vi "Filter Event Data.vi"(8 "error in (no error)":errorcluster, 10 "EventFilter Reference":T1, 11 "ListboxEditCellMsg In":refnum<class "ListboxEditCellMsg.lvclass">) -> (0 "error out":errorcluster, 2 "Discard?":bool, 3 "ListboxEditCellMsg Out":refnum<class "ListboxEditCellMsg.lvclass">)   [LabVIEW 2020, in "MVA Framework.lvlib" / "ActorEvents.lvlib" / "ListboxEditCellMsg.lvclass"]
uses:
  ListboxEditCellMsg.lvclass
  IEventFilter/EventFilter Reference.ctl
  IEventFilter/IEventFilter.lvclass
  ListboxEditCellMsg.lvclass/ListboxEditCellMsg.ctl
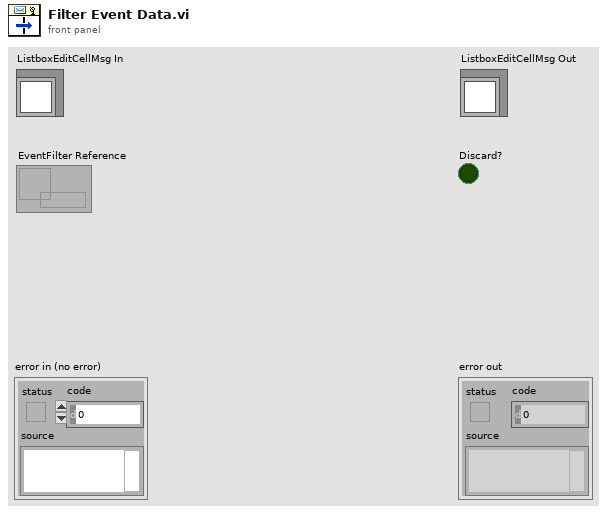
[diagram p1: front panel]
types:
  T1 = typedef "MVA Framework.lvlib/ActorEvents.lvlib/IEventFilter.lvclass/EventFilter Reference.ctl" = refnum<data-value>
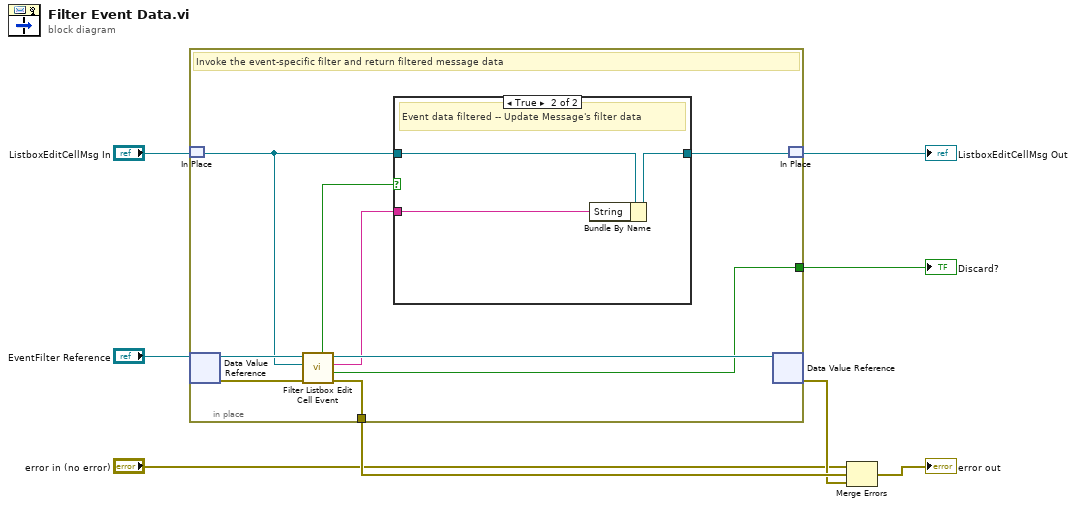
[diagram p0: block diagram]
diagram:
  n1 = in-place {
    in-place-border: [w13] -> w8
    in-place-border: [w14] -> w3
    # "Invoke the event-specific filter and return filtered message data"
    n2 = in-place-match #1("ListboxEditCellMsg In") -> (w11:refnum<class "ListboxEditCellMsg.lvclass">)
    n3 = in-place-dvr #2("EventFilter Reference") -> (w17:refnum<class "IEventFilter.lvclass">, w15:errorcluster)
    n4 = call-dynamic "Filter Listbox Edit Cell Event.vi"("error in (no error)"=w15, "ListboxEditCellMsg"=w11, "IEventFilter in"=w17) -> ("error out"=w13:errorcluster, "Discard?"=w14:bool, "Filtered String"=w12:string, "IEventFilter out"=w16:refnum<class "IEventFilter.lvclass">, "Data Filtered?"=w10:bool)  [unwired: 4 in]
    n5 = case shown="True" w10 {
      tunnel: w12 -> [_ w19]
      tunnel: w11 -> [w18 w21]
      tunnel: [w18 w20] -> w9
      frame False {
        # "No data filtered"
      }
      frame True {
        # "Event data filtered -- Update Message's filter data"
        n6 = Bundle By Name(cluster=w21, "String"=w19) -> (w20:refnum<class "ListboxEditCellMsg.lvclass">)
      }
    }
    n7 = in-place-dvr #2(w16) -> (w7:errorcluster)  [unwired: 1 out]
    n8 = in-place-match #1(w9) -> (→"ListboxEditCellMsg Out":refnum<class "ListboxEditCellMsg.lvclass">)
  }
  "Discard?" <- w3
  n9 = Merge Errors("error in (no error)", w8, w7) -> (→"error out":errorcluster)
